vi "Settings.Create.vi"(8 "error in (no error)":errorcluster, 10 "Type":T1, 11 "nodeID in":u64) -> (0 "error out":errorcluster, 3 "nodeID out":u64)   [LabVIEW 2019, in "Diagnostics Addon System Explorer.lvlib"]
uses:
  Diagnostics Addon System Explorer.lvlib
  Shared/Types/Type.ctl
  Shared/SubVIs/Constants.vi
  <vilib>/NI/NI VeriStand Advanced SysDef API/SysDef API/Advanced System Definition.lvlib
  Shared/Diagnostics Addon Shared.lvlib
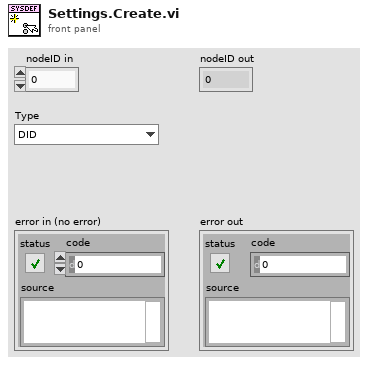
[diagram p1: front panel]
types:
  T1 = typedef "Diagnostics Addon Shared.lvlib/Type.ctl" = enum16{"DID", "CDID", "PID", "CPID", "Read Memory", "Write Memory", "IO Control", "Routine Start", "Routine Request", "Routine Stop", "User Defined", "DTC Control", "Clear DTCs", "Read DTCs", "Start DTCs", "DTC Change Count", "Tester Present", "Unlock ECU", "Reset ECU", "Diag Session Control", "Communication Control", "DPID Control", "Poll Control", "Diag CAN Control"}
  T2 = typedef "Diagnostics Addon Shared.lvlib/Protocol.ctl" = enum16{"GMLAN", "KWP-2000", "UDS", "User-Defined"}
  T3 = typedef "Custom Device API.lvlib/Custom Device Item Ref.ctl" = u64
  T4 = typedef "Diagnostics Addon System Explorer.lvlib/Settings.Channel.ctl" = cluster{"Name":string, "Channel":T5}
  T5 = typedef "Custom Device API.lvlib/Custom Device Channel.ctl" = cluster{"Type":T6, "Units":string, "Default Value":dbl, "Faultable":bool, "Scalable":bool}
  T6 = typedef "Custom Device API.lvlib/Custom Device Channel Type.ctl" = enum16{"Input", "Output"}
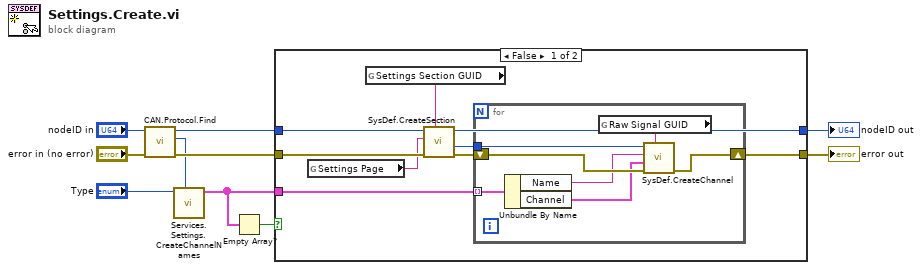
[diagram p0: block diagram]
diagram:
  n1 = call "CAN.Protocol.Find.vi"("error in (no error)"="error in (no error)", "Node Ptr"="nodeID in") -> ("error out"=w6:errorcluster, "Diagnostic Protocol"=w3:T2, "Section Ref out"=w4:T3)  [unwired: 7 in]
  n2 = call "Services.Settings.CreateChannelNames.vi"("Diagnostic Protocol"=w3, "Type"="Type") -> ("Settings Channels"=w10:T4[])  [unwired: 9 in]
  n3 = Empty Array?(array=w10) -> (empty?=w9:bool)
  n4 = case shown="False" w9 {
    tunnel: [w14 w28] -> w1
    tunnel: w4 -> [w18 w28]
    tunnel: [w15 w27] -> w2
    tunnel: w6 -> [w19 w27]
    tunnel: w10 -> [w13 _]
    frame False {
      n5 = global read "Constants.vi" "Settings Page"() -> (w11:string)
      n6 = global read "Constants.vi" "Settings Section GUID"() -> (w12:string)
      n7 = call <vilib>:"SysDef.CreateSection.vi"("GUID"=w12, "error in (no error)"=w19, "Name"=w11, "nodeID"=w18) -> ("error out"=w17:errorcluster, "New NodeID"=w16:u64, "nodeID out"=w14:u64)  [unwired: 4 in, 1 out]
      n8 = for {
        tunnel: w16 -> [w24]
        shift-right: [w23] -> w15
        shift-left: w17 -> [w25]
        tunnel: w13 -> [w22] mode=indexing
        n9 = Unbundle By Name(w22) -> ("Name"=w21:string, "Channel"=w20:T5)
        n10 = global read "Constants.vi" "Raw Signal GUID"() -> (w26:string)
        n11 = call <vilib>:"SysDef.CreateChannel.vi"("GUID"=w26, "error in (no error)"=w25, "Channel"=w20, "Name"=w21, "nodeID"=w24) -> ("error out"=w23:errorcluster)  [unwired: 3 in, 3 out]
      }
    }
    frame True {
    }
  }
  "error out" <- w2
  "nodeID out" <- w1
